vi "Main.vi"(8 "error in (no error)":errorcluster, 11 "DAQMH121119OrcaFlashBase in":refnum<class "DAQOrcaFlash.lvclass">) -> (0 "error out":errorcluster, 3 "component":refnum<class "DAQOrcaFlash.lvclass">)   [LabVIEW 2012, in "DAQOrcaFlash.lvclass"]
doc: "Main VI of the component."
uses:
  DAQOrcaFlash.lvclass
  binning.ctl
  visualisation_line_cluster.ctl
  merit_factor_type.ctl
  DAQOrcaFlash.lvclass/DAQOrcaFlash.ctl
  <vilib>/Distrio/Murmex/InitialiseMessage/InitialiseMessage.lvclass
  <vilib>/Distrio/Murmex/Murmex/command_enum.ctl
  <vilib>/Distrio/Murmex/TerminateMessage/TerminateMessage.lvclass
  <vilib>/Distrio/Murmex/StartMessage/StartMessage.lvclass
  <vilib>/Distrio/Murmex/StartMessage/run mode enum.ctl
  <vilib>/Distrio/Murmex/StopMessage/StopMessage.lvclass
  <vilib>/Distrio/Murmex/ConfigureMessage/ConfigureMessage.lvclass
  <vilib>/Distrio/Murmex/Murmex/update_cluster.ctl
  class variable.vi
  <vilib>/Distrio/Murmex/Murmex/Set VI reference.vi
  <vilib>/Distrio/Murmex/Murmex/Set configure at initialise.vi
  <vilib>/Distrio/Murmex/Murmex/Set relay start stop to observers.vi
  <vilib>/Distrio/Murmex/Murmex/Set log reference.vi
  <vilib>/Distrio/Murmex/Murmex/Set write log to disk.vi
  <vilib>/Distrio/Murmex/Murmex/Murmex.lvclass
  <vilib>/Distrio/Murmex/Message/Message.lvclass
panel:
  in  "button:configure":bool
  in  "button:quit":bool
  in  "terminate?":bool
  out "progress bar":sgl(slide) scale=0.0..1.0
  in  "Tab":T1(tab)
  in  "Rolling shutter pace":sgl[unit]=9.74436e-06 min=9.74436e-06 max=10 step=3.76e-09 format="%#_7g"
  out "Frames per second":dbl[unit]
  out "Virtual slit width":dbl[unit]
  in  "button:start_sweep":bool
  in  "y offset":u16 max=2048 step=4
  in  "x offset":u16 max=2048 step=4
  in  "y resolution":u16=2048 min=4 max=2048 step=4
  in  "x resolution":u16=2048 min=4 max=2048 step=4
  in  "binning":T2=1 items=["1x1"=1, "2x2"=2, "4x4"=4]
  in  "no. of frames":i32=1 min=1 step=1
  in  "line exposure time":dbl[unit]=0.1 caption="exposure time" min=9.700000000000001e-09 max=0.01
  in  "button:start focus":bool
  in  "wait b4 acquisition":dbl[unit]
  in  "file name":string
  in  "subfolder levels":string[](array[string])
  in  "Custom saving path":bool
  in  "directory out":path
  in  "button:convert":bool
  out "filename":string
  in  "directory in":path
  in  "ID":string="orca"
  in  "log":string
  out "time interval between MF":dbl
  out "Merit Factor":dbl
  in  "Merit factor type":T3
  in  "button:AO":bool
  in  "lines":T4[](array[typedef])
  in  "Conversion policy":T5={"Conversion Method"=10, "Minimum Value"=0, "Maximum Value"=0, "# Shifts"=0} {"Conversion Method" items=["Default"=10, "Most Significant Bits"=11, "Full Dynamic"=12, "Downshift"=13, "Given Range"=14, "90% Dynamic"=15, "Given Percent Range"=16]}
  # "Convert here properietary file formats of Hamamatsu to TIFF format."
  # "DAQOrcaFlash\n\nImplemented by:\nMarcel van 't Hoff\nLudovico Silvestri\nUniversity of Florence, Ital\n\nThis component supports only the Hamamatsu Orca Flash 4.0"
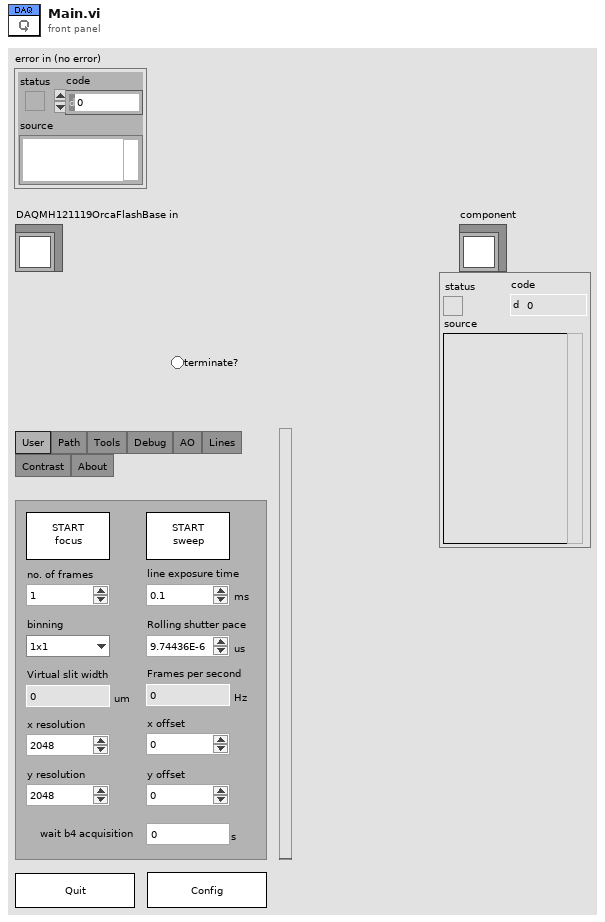
[diagram p1: front panel]
types:
  T1 = enum32{"User", "Path", "Tools", "Debug", "AO", "Lines", "Contrast", "About"}
  T2 = typedef "DAQOrcaFlash.lvclass/binning.ctl" = u16
  T3 = typedef "DAQOrcaFlash.lvclass/merit_factor_type.ctl" = enum16{"full frame intensity", "ROI beads", "Weber contrast", "Michelson contrast", "RMS contrast", "Line profile analysis", "ROI analysis", "FFT", "SNR", "5% brightest"}
  T4 = typedef "DAQOrcaFlash.lvclass/visualisation_line_cluster.ctl" = cluster{"direction":enum16{"horizontal", "vertical"}, "position":i32}
  T5 = cluster{"Conversion Method":u32, "Minimum Value":i32, "Maximum Value":i32, "# Shifts":i32}
  T6 = typedef "Murmex.lvlib/Murmex.lvclass/command_enum.ctl" = enum16{"null", "initialise", "reset", "terminate", "acknowledge", "update", "inspect", "inform", "proceed", "start", "stop", "fetch", "configure", "generic"}
  T7 = typedef "Murmex.lvlib/StartMessage.lvclass/run mode enum.ctl" = enum16{"infinite", "finite"}
  T8 = typedef "Murmex.lvlib/Murmex.lvclass/update_cluster.ctl" = cluster{"target ID":string, "key chains":string[], "values":variant[]}
  T9 = enum8{"Enabled", "Disabled", "Disabled and Grayed Out"}
  T10 = typedef "Murmex.lvclass/command_enum.ctl" = enum16{"null", "initialise", "reset", "terminate", "acknowledge", "update", "inspect", "inform", "proceed", "start", "stop", "fetch", "configure", "generic"}
  T11 = typedef "Murmex.lvclass/Event type enumerations.ctl" = enum16{"before", "after"}
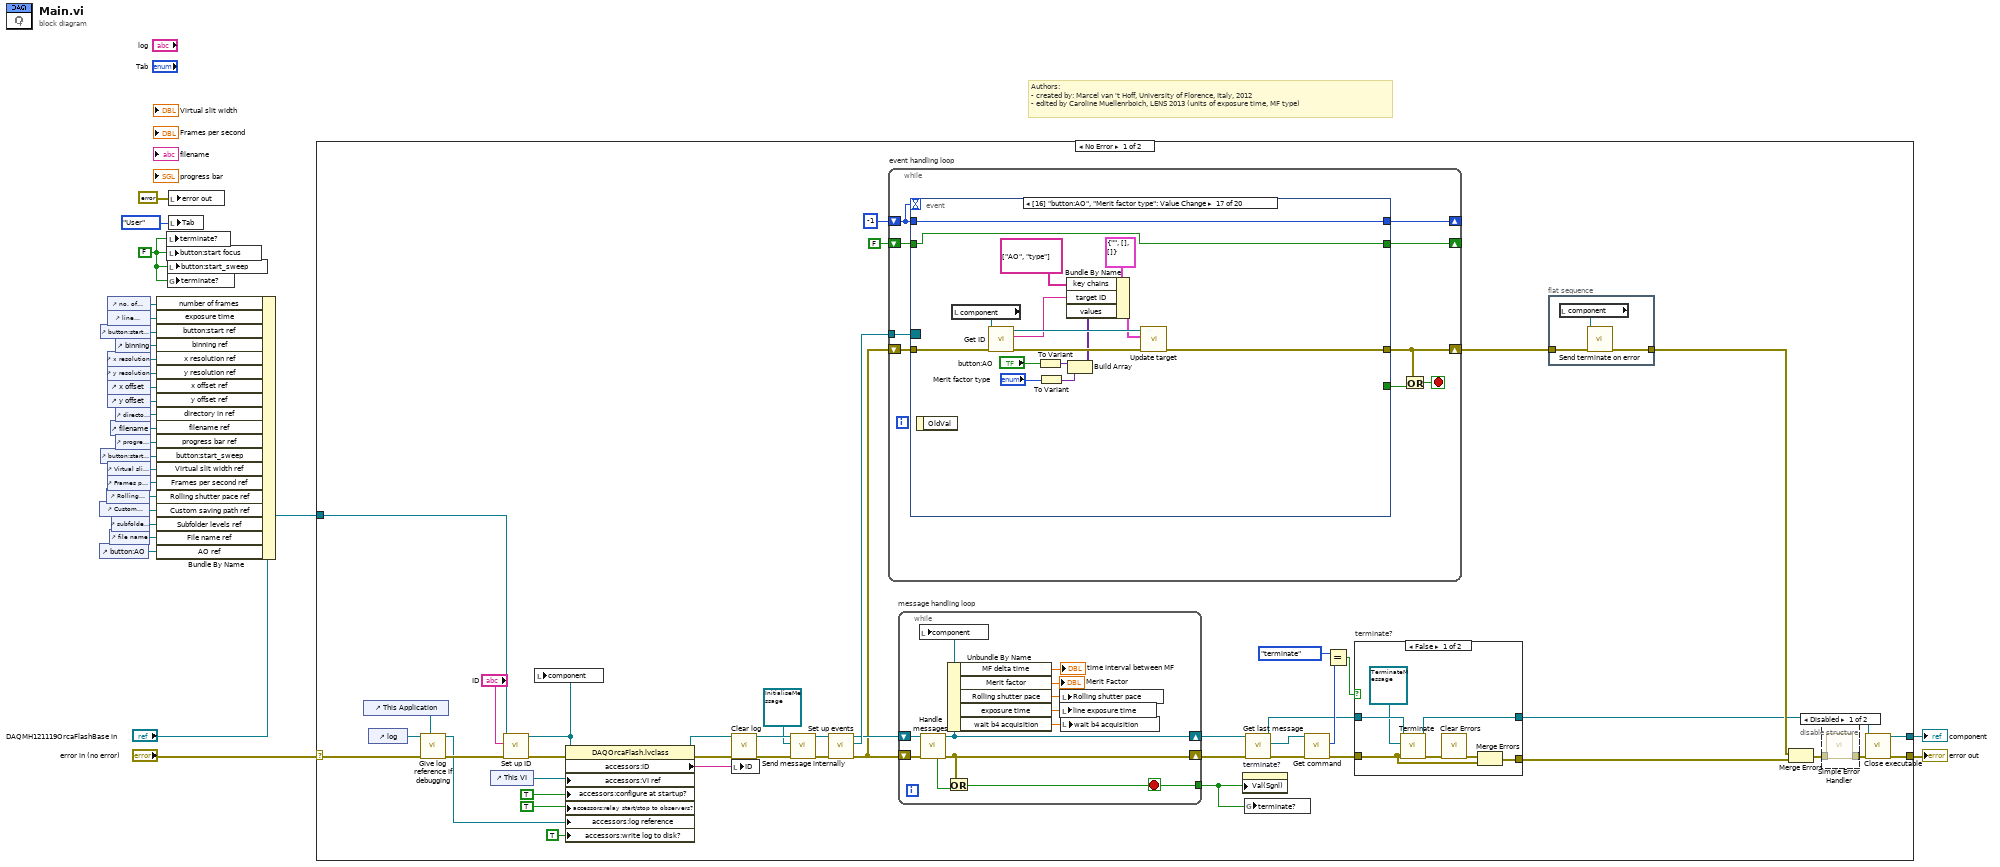
[diagram p0: block diagram]
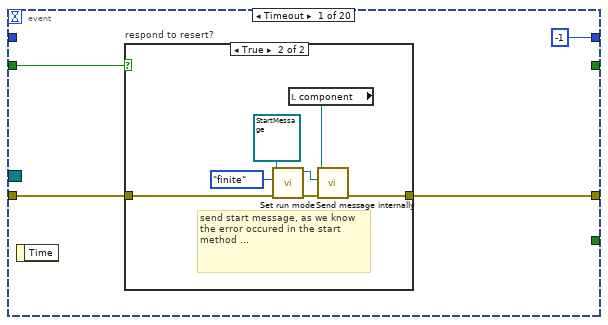
[diagram p4: hidden frame]
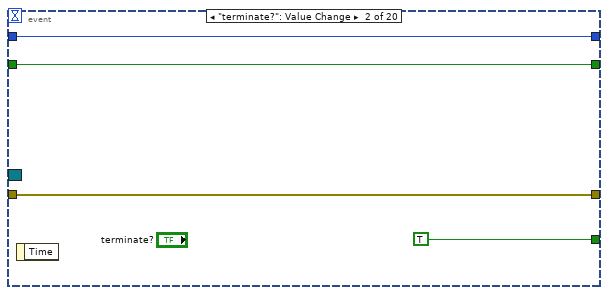
[diagram p6: hidden frame]
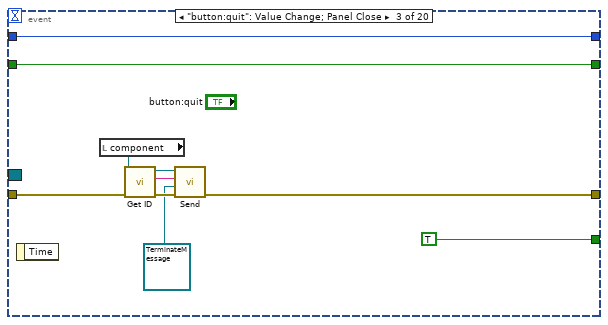
[diagram p7: hidden frame]
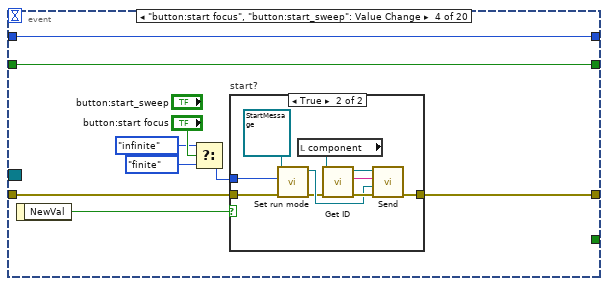
[diagram p8: hidden frame]
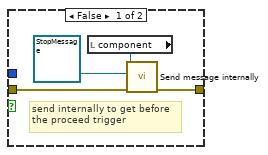
[diagram p9: hidden frame]
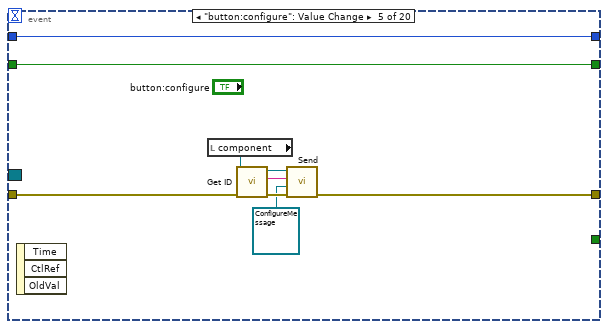
[diagram p10: hidden frame]
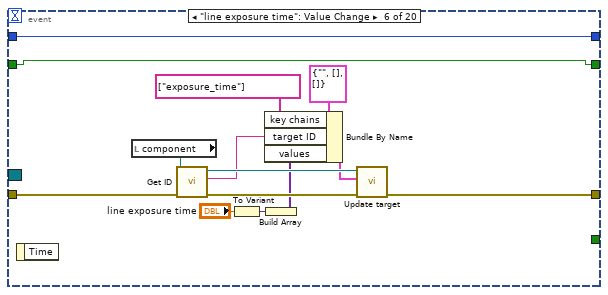
[diagram p11: hidden frame]
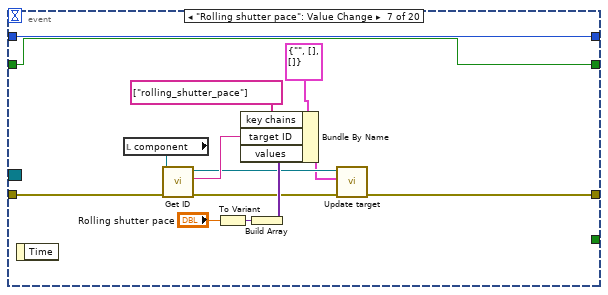
[diagram p12: hidden frame]
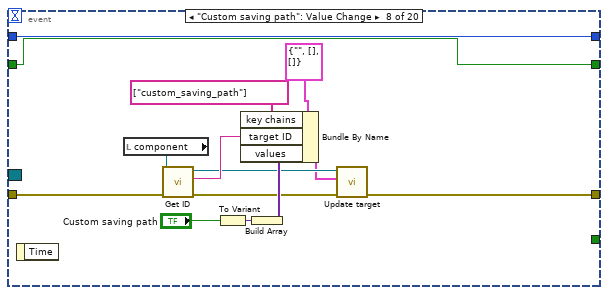
[diagram p13: hidden frame]
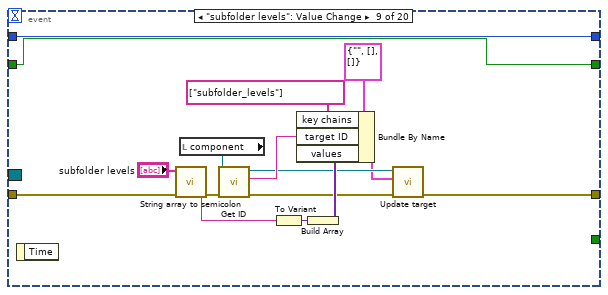
[diagram p14: hidden frame]
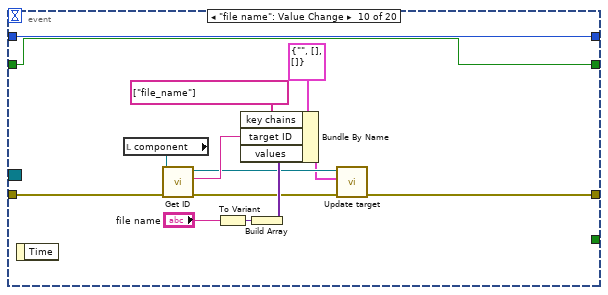
[diagram p15: hidden frame]
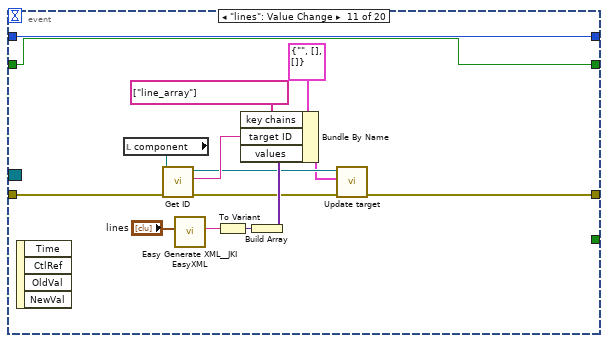
[diagram p16: hidden frame]
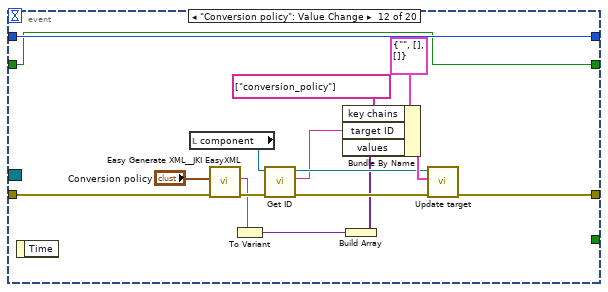
[diagram p17: hidden frame]
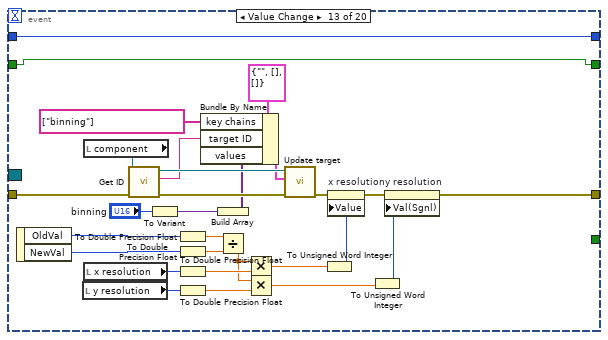
[diagram p18: hidden frame]
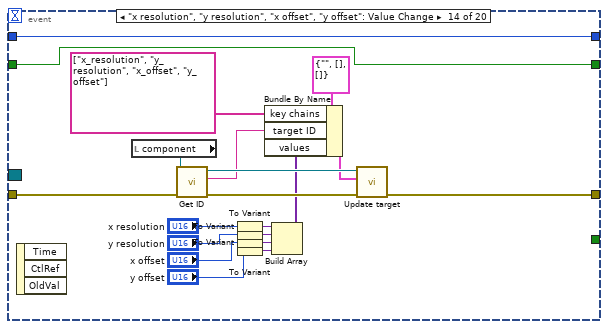
[diagram p19: hidden frame]
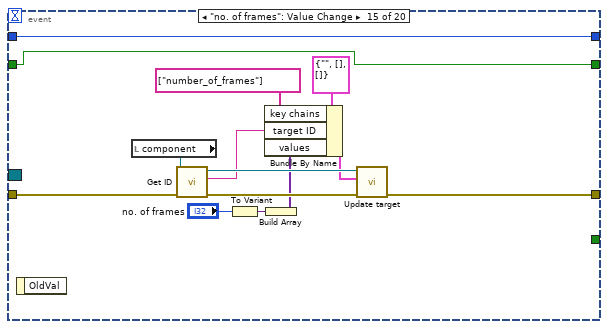
[diagram p20: hidden frame]
diagram:
  w9 = FALSE ("terminate?")
  # "Authors: \n- created by: Marcel van 't Hoff, University of Florence, Italy, 2012\n- edited by Caroline Muellenrboich, LENS 2013 (units of exposure time, MF type)"
  n1 = control-ref of="button:AO"() -> (w2:refnum<vi>)
  n2 = control-ref of="Custom saving path"() -> (w3:refnum<vi>)
  n3 = control-ref of="button:start focus"() -> (w20:refnum<vi>)
  n4 = control-ref of="button:start_sweep"() -> (w10:refnum<vi>)
  n5 = control-ref of="Rolling shutter pace"() -> (w6:refnum<vi>)
  n6 = control-ref of="no. of frames"() -> (w21:refnum<vi>)
  n7 = control-ref of="line exposure time"() -> (w22:refnum<vi>)
  n8 = control-ref of="x resolution"() -> (w18:refnum<vi>)
  n9 = control-ref of="y resolution"() -> (w17:refnum<vi>)
  n10 = control-ref of="x offset"() -> (w16:refnum<vi>)
  n11 = control-ref of="y offset"() -> (w15:refnum<vi>)
  n12 = control-ref of="Virtual slit width"() -> (w8:refnum<vi>)
  n13 = control-ref of="Frames per second"() -> (w7:refnum<vi>)
  n14 = control-ref of="file name"() -> (w5:refnum<vi>)
  n15 = control-ref of="filename"() -> (w13:refnum<vi>)
  n16 = control-ref of="subfolder levels"() -> (w4:refnum<vi>)
  n17 = control-ref of="binning"() -> (w19:refnum<vi>)
  n18 = control-ref of="directory in"() -> (w14:refnum<vi>)
  n19 = control-ref of="progress bar"() -> (w12:refnum<vi>)
  n20 = Bundle By Name(cluster="DAQMH121119OrcaFlashBase in", "number of frames"=w21, "exposure time"=w22, "button:start ref"=w20, "binning ref"=w19, "x resolution ref"=w18, "y resolution ref"=w17, "x offset ref"=w16, "y offset ref"=w15, "directory in ref"=w14, "filename ref"=w13, "progress bar ref"=w12, "button:start_sweep"=w10, "Virtual slit width ref"=w8, "Frames per second ref"=w7, "Rolling shutter pace ref"=w6, "Custom saving path ref"=w3, "Subfolder levels ref"=w4, "File name ref"=w5, "AO ref"=w2) -> (w23:refnum<class "DAQOrcaFlash.lvclass">)
  n21 = local write "terminate?"(w9) -> ()
  n22 = local write "button:start focus"(w9) -> ()
  n23 = local write "button:start_sweep"(w9) -> ()
  n24 = global write "class variable.vi" "terminate?"(w9) -> ()
  n25 = local write "error out"(errorcluster {"status"=FALSE, "code"=0, "source"=""} ("error out")) -> ()
  n26 = local write "Tab"(T1."User" ("Tab")) -> ()
  n27 = case shown="No Error" "error in (no error)" {
    selector: "error in (no error)" -> [w34 w437]
    tunnel: [w61 w437] -> w26
    tunnel: [w60 w436] -> w25
    tunnel: w23 -> [w66 w436]
    frame No Error {
      n28 = control-ref of="This Application"() -> (w30:refnum<vi>)
      n29 = control-ref of="log"() -> (w32:refnum<vi>)
      n30 = call "Give log reference if debugging.vi"("application ref"=w30, "error in (no error)"=w34, "log reference in"=w32) -> ("error out"=w33:errorcluster, "log reference out"=w31:refnum<vi>)  [unwired: 6 in, 1 out]
      n31 = control-ref of="This VI"() -> (w56:refnum<vi>)
      n32 = call <vilib>:"Set up ID.vi"("error in (no error)"=w33, "component ID"="ID", "MurmexBase in"=w66) -> ("error out"=w58:errorcluster, "MurmexBase out"=w47:refnum<class "DAQOrcaFlash.lvclass">)  [unwired: 6 in, 1 out]
      n33 = local write "component"(w47) -> ()
      n34 = property class="DAQOrcaFlash.lvclass"(reference=w47, error in=w58, "accessors:VI ref"=w56, "accessors:configure at startup?"=TRUE ("configure at startup?"), "accessors:relay start/stop to observers?"=TRUE ("relay start/stop to observers?"), "accessors:log reference"=w31, "accessors:write log to disk?"=TRUE ("write log to disk?")) -> (reference out=w54:refnum<class "DAQOrcaFlash.lvclass">, error out=w55:errorcluster, "accessors:ID"=w57:string)
      n35 = call <vilib>:"Clear log.vi"("error in (no error)"=w55, "MurmexBase in"=w54) -> ("error out"=w67:errorcluster, "MurmexBase out"=w71:refnum<class "DAQOrcaFlash.lvclass">)  [unwired: 8 in]
      n36 = local write "ID"(w57) -> ()
      n37 = call <vilib>:"Send message internally.vi"("error in (no error)"=w67, "Message"=refnum<class "InitialiseMessage.lvclass"> refnum ("Distrio Murmex 1.0:InitialiseMessage"), "Murmex in"=w71) -> ("error out"=w64:errorcluster, "Murmex out"=w63:refnum<class "DAQOrcaFlash.lvclass">)  [unwired: 7 in]
      n38 = call <vilib>:"Set up events.vi"("error in (no error)"=w64, "MurmexBase in"=w63) -> ("error out"=w36:errorcluster, "Event Registration Refnum"=w69:refnum<event-registration>, "MurmexBase out"=w38:refnum<class "DAQOrcaFlash.lvclass">)  [unwired: 7 in]
      n39 = while "event handling loop" {
        shift-right: [w94] -> _
        shift-left: -1 -> [w93]
        tunnel: w69 -> [w91]
        shift-right: [w90] -> w68
        shift-left: w36 -> [w92]
        shift-right: [w87] -> _
        shift-left: FALSE ("respond to reset?") -> [w86]
        stop <- w88 stop-if-true
        n40 = event shown="[16] \"button:AO\", \"Merit factor type\": Value Change" {
          selector: w91 -> [_ _ _ _ _ _ _ _ _ _ _ _ _ _ _ _ _ _ _ _]
          dyn-events: _ -> [_ _ _ _ _ _ _ _ _ _ _ _ _ _ _ _ _ _ _ _]
          timeout: w93 -> [_ _ _ _ _ _ _ _ _ _ _ _ _ _ _ _ _ _ _ _]
          tunnel: [-1 w110 w120 w129 w152 w166 w180 w194 w210 w224 w239 w255 w284 w304 w318 w332 w348 w350 w412 w424] -> w94
          tunnel: w93 -> [_ w110 w120 w129 w152 w166 w180 w194 w210 w224 w239 w255 w284 w304 w318 w332 w348 w355 w412 w424]
          tunnel: w92 -> [w96 w109 w113 w128 w148 w165 w179 w193 w199 w223 w238 w254 w283 w303 w317 w331 w347 w356 w410 w421]
          tunnel: [w95 w109 w115 w127 w147 w164 w172 w182 w203 w216 w231 w249 w266 w302 w316 w330 w336 w357 w409 w414] -> w90
          tunnel: [_ TRUE TRUE _ _ _ _ _ _ _ _ _ _ _ _ _ _ _ _ _] -> w89
          tunnel: [_ w107 w111 w121 w144 w153 w167 w181 w195 w211 w225 w240 w256 w285 w305 w319 w335 w352 w406 w413] -> w87
          tunnel: w86 -> [w97 w107 w111 w121 w144 w153 w167 w181 w195 w211 w225 w240 w256 w285 w305 w319 w335 w353 w406 w413]
          event Timeout {
            n41 = event-data() -> ()  [unwired: 1 in, 1 out]
            n42 = case "respond to resert?" shown="True" w97 {
              tunnel: w96 -> [w99 w102]
              tunnel: [w99 w106] -> w95
              frame False {
              }
              frame True {
                # "send start message, as we know the error occured in the start method ..."
                n43 = call <vilib>:"Set run mode.vi"("error in (no error)"=w102, "run mode"=run_mode_enum."finite", "StartMessage in"=refnum<class "StartMessage.lvclass"> refnum ("Distrio Murmex 1.0:StartMessage")) -> ("error out"=w101:errorcluster, "StartMessage out"=w103:refnum<class "StartMessage.lvclass">)  [unwired: 7 in]
                n44 = local read "component"() -> (w105:refnum<class "DAQOrcaFlash.lvclass">)
                n45 = call <vilib>:"Send message internally.vi"("error in (no error)"=w101, "Message"=w103, "Murmex in"=w105) -> ("error out"=w106:errorcluster)  [unwired: 7 in, 1 out]
              }
            }
          }
          event "terminate?": Value Change {
            n46 = event-data() -> ()  [unwired: 1 in, 1 out]
          }
          event "button:quit": Value Change; Panel Close {
            n47 = event-data() -> ()  [unwired: 1 in, 1 out]
            n48 = local read "component"() -> (w118:refnum<class "DAQOrcaFlash.lvclass">)
            n49 = call <vilib>:"Get ID.vi"("error in (no error)"=w113, "Murmex in"=w118) -> ("error out"=w114:errorcluster, "component id"=w116:string, "Murmex out"=w117:refnum<class "DAQOrcaFlash.lvclass">)  [unwired: 7 in]
            n50 = call <vilib>:"Send.vi"("error in (no error)"=w114, "Message"=refnum<class "TerminateMessage.lvclass"> refnum ("Message in"), "recipient"=w116, "Murmex in"=w117) -> ("error out"=w115:errorcluster)  [unwired: 6 in, 1 out]
          }
          event "button:start focus", "button:start_sweep": Value Change {
            n51 = event-data() -> ("NewVal"=w124:bool)  [unwired: 1 in]
            n52 = Select(t=run_mode_enum."infinite" ("run mode"), s="button:start focus", f=run_mode_enum."finite" ("run mode")) -> (s? t:f=w125:T7)
            n53 = case "start?" shown="True" w124 {
              tunnel: [w132 w139] -> w127
              tunnel: w128 -> [w133 w136]
              tunnel: w125 -> [_ w134]
              frame False {
                # "send internally to get before\nthe proceed trigger"
                n54 = local read "component"() -> (w131:refnum<class "DAQOrcaFlash.lvclass">)
                n55 = call <vilib>:"Send message internally.vi"("error in (no error)"=w133, "Message"=refnum<class "StopMessage.lvclass"> refnum ("Distrio Murmex 1.0:StopMessage"), "Murmex in"=w131) -> ("error out"=w132:errorcluster)  [unwired: 7 in, 1 out]
              }
              frame True {
                n56 = call <vilib>:"Set run mode.vi"("error in (no error)"=w136, "run mode"=w134, "StartMessage in"=refnum<class "StartMessage.lvclass"> refnum ("Distrio Murmex 1.0:StartMessage")) -> ("error out"=w135:errorcluster, "StartMessage out"=w137:refnum<class "StartMessage.lvclass">)  [unwired: 7 in]
                n57 = local read "component"() -> (w143:refnum<class "DAQOrcaFlash.lvclass">)
                n58 = call <vilib>:"Get ID.vi"("error in (no error)"=w135, "Murmex in"=w143) -> ("error out"=w140:errorcluster, "component id"=w141:string, "Murmex out"=w142:refnum<class "DAQOrcaFlash.lvclass">)  [unwired: 7 in]
                n59 = call <vilib>:"Send.vi"("error in (no error)"=w140, "Message"=w137, "recipient"=w141, "Murmex in"=w142) -> ("error out"=w139:errorcluster)  [unwired: 6 in, 1 out]
              }
            }
          }
          event "button:configure": Value Change {
            n60 = event-data() -> ()  [unwired: 1 in, 3 out]
            n61 = local read "component"() -> (w146:refnum<class "DAQOrcaFlash.lvclass">)
            n62 = call <vilib>:"Get ID.vi"("error in (no error)"=w148, "Murmex in"=w146) -> ("error out"=w149:errorcluster, "component id"=w150:string, "Murmex out"=w151:refnum<class "DAQOrcaFlash.lvclass">)  [unwired: 7 in]
            n63 = call <vilib>:"Send.vi"("error in (no error)"=w149, "Message"=refnum<class "ConfigureMessage.lvclass"> refnum ("ConfigureMessage"), "recipient"=w150, "Murmex in"=w151) -> ("error out"=w147:errorcluster)  [unwired: 6 in, 1 out]
          }
          event "line exposure time": Value Change {
            n64 = event-data() -> ()  [unwired: 1 in, 1 out]
            n65 = local read "component"() -> (w163:refnum<class "DAQOrcaFlash.lvclass">)
            n66 = call <vilib>:"Get ID.vi"("error in (no error)"=w165, "Murmex in"=w163) -> ("error out"=w161:errorcluster, "component id"=w158:string, "Murmex out"=w162:refnum<class "DAQOrcaFlash.lvclass">)  [unwired: 7 in]
            n67 = To Variant(anything="line exposure time") -> (Variant=w156:variant)
            n68 = Build Array(w156) -> (w155:variant[])
            n69 = Bundle By Name(cluster=T8 {"target ID"="", "key chains"=[], "values"=[]} ("update cluster"), "key chains"=string[] ["exposure_time"], "target ID"=w158, "values"=w155) -> (w159:T8)
            n70 = call <vilib>:"Update target.vi"("error in (no error)"=w161, "update cluster"=w159, "MurmexBase in"=w162) -> ("error out"=w164:errorcluster)  [unwired: 7 in, 1 out]
          }
          event "Rolling shutter pace": Value Change {
            n71 = event-data() -> ()  [unwired: 1 in, 1 out]
            n72 = local read "component"() -> (w177:refnum<class "DAQOrcaFlash.lvclass">)
            n73 = call <vilib>:"Get ID.vi"("error in (no error)"=w179, "Murmex in"=w177) -> ("error out"=w173:errorcluster, "component id"=w176:string, "Murmex out"=w171:refnum<class "DAQOrcaFlash.lvclass">)  [unwired: 7 in]
            n74 = To Variant(anything="Rolling shutter pace") -> (Variant=w178:variant)
            n75 = Build Array(w178) -> (w174:variant[])
            n76 = Bundle By Name(cluster=T8 {"target ID"="", "key chains"=[], "values"=[]} ("update cluster"), "key chains"=string[] ["rolling_shutter_pace"], "target ID"=w176, "values"=w174) -> (w169:T8)
            n77 = call <vilib>:"Update target.vi"("error in (no error)"=w173, "update cluster"=w169, "MurmexBase in"=w171) -> ("error out"=w172:errorcluster)  [unwired: 7 in, 1 out]
          }
          event "Custom saving path": Value Change {
            n78 = event-data() -> ()  [unwired: 1 in, 1 out]
            n79 = local read "component"() -> (w191:refnum<class "DAQOrcaFlash.lvclass">)
            n80 = call <vilib>:"Get ID.vi"("error in (no error)"=w193, "Murmex in"=w191) -> ("error out"=w187:errorcluster, "component id"=w190:string, "Murmex out"=w186:refnum<class "DAQOrcaFlash.lvclass">)  [unwired: 7 in]
            n81 = To Variant(anything="Custom saving path") -> (Variant=w192:variant)
            n82 = Build Array(w192) -> (w188:variant[])
            n83 = Bundle By Name(cluster=T8 {"target ID"="", "key chains"=[], "values"=[]} ("update cluster"), "key chains"=string[] ["custom_saving_path"], "target ID"=w190, "values"=w188) -> (w184:T8)
            n84 = call <vilib>:"Update target.vi"("error in (no error)"=w187, "update cluster"=w184, "MurmexBase in"=w186) -> ("error out"=w182:errorcluster)  [unwired: 7 in, 1 out]
          }
          event "subfolder levels": Value Change {
            n85 = event-data() -> ()  [unwired: 1 in, 1 out]
            n86 = call "String array to semicolon.vi"("error in"=w199, "String array"="subfolder levels") -> ("error out"=w198:errorcluster, "Semicolon string"=w197:string)  [unwired: 8 in]
            n87 = local read "component"() -> (w208:refnum<class "DAQOrcaFlash.lvclass">)
            n88 = call <vilib>:"Get ID.vi"("error in (no error)"=w198, "Murmex in"=w208) -> ("error out"=w204:errorcluster, "component id"=w207:string, "Murmex out"=w202:refnum<class "DAQOrcaFlash.lvclass">)  [unwired: 7 in]
            n89 = To Variant(anything=w197) -> (Variant=w209:variant)
            n90 = Build Array(w209) -> (w205:variant[])
            n91 = Bundle By Name(cluster=T8 {"target ID"="", "key chains"=[], "values"=[]} ("update cluster"), "key chains"=string[] ["subfolder_levels"], "target ID"=w207, "values"=w205) -> (w200:T8)
            n92 = call <vilib>:"Update target.vi"("error in (no error)"=w204, "update cluster"=w200, "MurmexBase in"=w202) -> ("error out"=w203:errorcluster)  [unwired: 7 in, 1 out]
          }
          event "file name": Value Change {
            n93 = event-data() -> ()  [unwired: 1 in, 1 out]
            n94 = local read "component"() -> (w221:refnum<class "DAQOrcaFlash.lvclass">)
            n95 = call <vilib>:"Get ID.vi"("error in (no error)"=w223, "Murmex in"=w221) -> ("error out"=w217:errorcluster, "component id"=w220:string, "Murmex out"=w215:refnum<class "DAQOrcaFlash.lvclass">)  [unwired: 7 in]
            n96 = To Variant(anything="file name") -> (Variant=w222:variant)
            n97 = Build Array(w222) -> (w218:variant[])
            n98 = Bundle By Name(cluster=T8 {"target ID"="", "key chains"=[], "values"=[]} ("update cluster"), "key chains"=string[] ["file_name"], "target ID"=w220, "values"=w218) -> (w213:T8)
            n99 = call <vilib>:"Update target.vi"("error in (no error)"=w217, "update cluster"=w213, "MurmexBase in"=w215) -> ("error out"=w216:errorcluster)  [unwired: 7 in, 1 out]
          }
          event "lines": Value Change {
            n100 = event-data() -> ()  [unwired: 1 in, 4 out]
            n101 = local read "component"() -> (w236:refnum<class "DAQOrcaFlash.lvclass">)
            n102 = call <vilib>:"Get ID.vi"("error in (no error)"=w238, "Murmex in"=w236) -> ("error out"=w232:errorcluster, "component id"=w235:string, "Murmex out"=w230:refnum<class "DAQOrcaFlash.lvclass">)  [unwired: 7 in]
            n103 = call <vilib>:"Easy Generate XML__JKI EasyXML.vi"("LabVIEW Data"="lines") -> ("XML String"=w226:string)  [unwired: 9 in, 1 out]
            n104 = To Variant(anything=w226) -> (Variant=w237:variant)
            n105 = Build Array(w237) -> (w233:variant[])
            n106 = Bundle By Name(cluster=T8 {"target ID"="", "key chains"=[], "values"=[]} ("update cluster"), "key chains"=string[] ["line_array"], "target ID"=w235, "values"=w233) -> (w228:T8)
            n107 = call <vilib>:"Update target.vi"("error in (no error)"=w232, "update cluster"=w228, "MurmexBase in"=w230) -> ("error out"=w231:errorcluster)  [unwired: 7 in, 1 out]
          }
          event "Conversion policy": Value Change {
            n108 = event-data() -> ()  [unwired: 1 in, 1 out]
            n109 = local read "component"() -> (w250:refnum<class "DAQOrcaFlash.lvclass">)
            n110 = call <vilib>:"Easy Generate XML__JKI EasyXML.vi"("error in (no error)"=w254, "LabVIEW Data"="Conversion policy") -> ("error out"=w253:errorcluster, "XML String"=w242:string)  [unwired: 8 in]
            n111 = To Variant(anything=w242) -> (Variant=w243:variant)
            n112 = call <vilib>:"Get ID.vi"("error in (no error)"=w253, "Murmex in"=w250) -> ("error out"=w251:errorcluster, "component id"=w244:string, "Murmex out"=w245:refnum<class "DAQOrcaFlash.lvclass">)  [unwired: 7 in]
            n113 = Build Array(w243) -> (w241:variant[])
            n114 = Bundle By Name(cluster=T8 {"target ID"="", "key chains"=[], "values"=[]} ("update cluster"), "key chains"=string[] ["conversion_policy"], "target ID"=w244, "values"=w241) -> (w246:T8)
            n115 = call <vilib>:"Update target.vi"("error in (no error)"=w251, "update cluster"=w246, "MurmexBase in"=w245) -> ("error out"=w249:errorcluster)  [unwired: 7 in, 1 out]
          }
          event Value Change {
            n116 = event-data() -> ("OldVal"=w261:T2, "NewVal"=w260:T2)  [unwired: 1 in]
            n117 = local read "y resolution"() -> (w274:u16)
            n118 = local read "component"() -> (w282:refnum<class "DAQOrcaFlash.lvclass">)
            n119 = local read "x resolution"() -> (w273:u16)
            n120 = call <vilib>:"Get ID.vi"("error in (no error)"=w283, "Murmex in"=w282) -> ("error out"=w280:errorcluster, "component id"=w277:string, "Murmex out"=w281:refnum<class "DAQOrcaFlash.lvclass">)  [unwired: 7 in]
            n121 = To Variant(anything="binning") -> (Variant=w269:variant)
            n122 = To Double Precision Float(number=w261) -> (double precision float=w259:dbl)
            n123 = To Double Precision Float(number=w260) -> (double precision float=w258:dbl)
            n124 = To Double Precision Float(number=w273) -> (double precision float=w270:dbl)
            n125 = To Double Precision Float(number=w274) -> (double precision float=w271:dbl)
            n126 = Build Array(w269) -> (w275:variant[])
            n127 = Bundle By Name(cluster=T8 {"target ID"="", "key chains"=[], "values"=[]} ("update cluster"), "key chains"=string[] ["binning"], "target ID"=w277, "values"=w275) -> (w278:T8)
            n128 = Divide(x=w259, y=w258) -> (x/y=w257:dbl)
            n129 = Multiply(x=w257, y=w270) -> (x*y=w267:dbl)
            n130 = Multiply(x=w257, y=w271) -> (x*y=w268:dbl)
            n131 = call <vilib>:"Update target.vi"("error in (no error)"=w280, "update cluster"=w278, "MurmexBase in"=w281) -> ("error out"=w265:errorcluster)  [unwired: 7 in, 1 out]
            n132 = To Unsigned Word Integer(number=w267) -> (unsigned 16bit integer=w264:u16)
            n133 = property on="x resolution" class="DigNum (strict)"(error in=w265, "Value"=w264) -> (error out=w262:errorcluster)  [unwired: 1 in, 1 out]
            n134 = To Unsigned Word Integer(number=w268) -> (unsigned 16bit integer=w263:u16)
            n135 = property on="y resolution" class="DigNum (strict)"(error in=w262, "Val(Sgnl)"=w263) -> (error out=w266:errorcluster)  [unwired: 1 in, 1 out]
          }
          event "x resolution", "y resolution", "x offset", "y offset": Value Change {
            n136 = event-data() -> ()  [unwired: 1 in, 3 out]
            n137 = local read "component"() -> (w301:refnum<class "DAQOrcaFlash.lvclass">)
            n138 = call <vilib>:"Get ID.vi"("error in (no error)"=w303, "Murmex in"=w301) -> ("error out"=w299:errorcluster, "component id"=w296:string, "Murmex out"=w300:refnum<class "DAQOrcaFlash.lvclass">)  [unwired: 7 in]
            n139 = To Variant(anything="x resolution") -> (Variant=w289:variant)
            n140 = To Variant(anything="y resolution") -> (Variant=w288:variant)
            n141 = To Variant(anything="x offset") -> (Variant=w287:variant)
            n142 = To Variant(anything="y offset") -> (Variant=w286:variant)
            n143 = Build Array(w289, w288, w287, w286) -> (w290:variant[])
            n144 = Bundle By Name(cluster=T8 {"target ID"="", "key chains"=[], "values"=[]} ("update cluster"), "key chains"=string[] ["x_resolution", "y_resolution", "x_offset", "y_offset"], "target ID"=w296, "values"=w290) -> (w297:T8)
            n145 = call <vilib>:"Update target.vi"("error in (no error)"=w299, "update cluster"=w297, "MurmexBase in"=w300) -> ("error out"=w302:errorcluster)  [unwired: 7 in, 1 out]
          }
          event "no. of frames": Value Change {
            n146 = event-data() -> ()  [unwired: 1 in, 1 out]
            n147 = local read "component"() -> (w315:refnum<class "DAQOrcaFlash.lvclass">)
            n148 = call <vilib>:"Get ID.vi"("error in (no error)"=w317, "Murmex in"=w315) -> ("error out"=w313:errorcluster, "component id"=w310:string, "Murmex out"=w314:refnum<class "DAQOrcaFlash.lvclass">)  [unwired: 7 in]
            n149 = To Variant(anything="no. of frames") -> (Variant=w306:variant)
            n150 = Build Array(w306) -> (w308:variant[])
            n151 = Bundle By Name(cluster=T8 {"target ID"="", "key chains"=[], "values"=[]} ("update cluster"), "key chains"=string[] ["number_of_frames"], "target ID"=w310, "values"=w308) -> (w311:T8)
            n152 = call <vilib>:"Update target.vi"("error in (no error)"=w313, "update cluster"=w311, "MurmexBase in"=w314) -> ("error out"=w316:errorcluster)  [unwired: 7 in, 1 out]
          }
          event "wait b4 acquisition": Value Change {
            # "waitb4 is a fun name for a control, but do you really need\nto use this also for the settings?"
            n153 = event-data() -> ()  [unwired: 1 in, 1 out]
            n154 = local read "component"() -> (w329:refnum<class "DAQOrcaFlash.lvclass">)
            n155 = call <vilib>:"Get ID.vi"("error in (no error)"=w331, "Murmex in"=w329) -> ("error out"=w327:errorcluster, "component id"=w324:string, "Murmex out"=w328:refnum<class "DAQOrcaFlash.lvclass">)  [unwired: 7 in]
            n156 = To Variant(anything="wait b4 acquisition") -> (Variant=w321:variant)
            n157 = Build Array(w321) -> (w322:variant[])
            n158 = Bundle By Name(cluster=T8 {"target ID"="", "key chains"=[], "values"=[]} ("update cluster"), "key chains"=string[] ["waitb4"], "target ID"=w324, "values"=w322) -> (w325:T8)
            n159 = call <vilib>:"Update target.vi"("error in (no error)"=w327, "update cluster"=w325, "MurmexBase in"=w328) -> ("error out"=w330:errorcluster)  [unwired: 7 in, 1 out]
          }
          event "button:AO": Value Change {
            n160 = event-data() -> ()  [unwired: 1 in, 1 out]
            n161 = local read "component"() -> (w346:refnum<class "DAQOrcaFlash.lvclass">)
            n162 = call <vilib>:"Get ID.vi"("error in (no error)"=w347, "Murmex in"=w346) -> ("error out"=w344:errorcluster, "component id"=w337:string, "Murmex out"=w345:refnum<class "DAQOrcaFlash.lvclass">)  [unwired: 7 in]
            n163 = To Variant(anything="button:AO") -> (Variant=w339:variant)
            n164 = To Variant(anything="Merit factor type") -> (Variant=w334:variant)
            n165 = Build Array(w339, w334) -> (w340:variant[])
            n166 = Bundle By Name(cluster=T8 {"target ID"="", "key chains"=[], "values"=[]} ("update cluster"), "key chains"=string[] ["AO", "type"], "target ID"=w337, "values"=w340) -> (w342:T8)
            n167 = call <vilib>:"Update target.vi"("error in (no error)"=w344, "update cluster"=w342, "MurmexBase in"=w345) -> ("error out"=w336:errorcluster)  [unwired: 7 in, 1 out]
          }
          event User Event {
            w349 = 5000  # wait for starting
            n168 = event-data() -> ("command"=w358:T10, "event type"=w354:T11)  [unwired: 1 in]
            n169 = case "command?" shown="\"reset\"" w358 {
              tunnel: [w363 w375 w387 w402 w405] -> w357
              tunnel: w356 -> [w362 w374 w388 w402 w405]
              tunnel: [w361 w373 w386 w400 w404] -> w351
              tunnel: w355 -> [w361 w373 w385 w400 w404]
              tunnel: w354 -> [w360 w372 w384 _ _]
              tunnel: [w359 w371 w383 w401 w403] -> w352
              tunnel: w353 -> [w359 w371 w383 _ w403]
              frame "stop" {
                n170 = case shown="\"after\"" w360 {
                  tunnel: [w364 w370] -> w363
                  tunnel: w362 -> [w364 w367]
                  frame "before", Default {
                  }
                  frame "after" {
                    n171 = local read "component"() -> (w368:refnum<class "DAQOrcaFlash.lvclass">)
                    n172 = call "Get GUI refs.vi"("error in (no error)"=w367, "DAQMH121119OrcaFlash in"=w368) -> ("error out"=w366:errorcluster, "Array"=w365:refnum<vi>[])  [unwired: 7 in, 1 out]
                    n173 = call <vilib>:"Disable GUI elements.vi"("error in (no error)"=w366, "enabled state"=T9."Enabled", "control refs"=w365) -> ("error out"=w370:errorcluster)  [unwired: 8 in]
                  }
                }
              }
              frame "start" {
                n174 = case shown="\"after\"" w372 {
                  tunnel: [w376 w382] -> w375
                  tunnel: w374 -> [w376 w380]
                  frame "before", Default {
                  }
                  frame "after" {
                    n175 = local read "component"() -> (w377:refnum<class "DAQOrcaFlash.lvclass">)
                    n176 = call "Get GUI refs.vi"("error in (no error)"=w380, "DAQMH121119OrcaFlash in"=w377) -> ("error out"=w379:errorcluster, "Array"=w378:refnum<vi>[])  [unwired: 7 in, 1 out]
                    n177 = call <vilib>:"Disable GUI elements.vi"("error in (no error)"=w379, "enabled state"=T9."Disabled and Grayed Out", "control refs"=w378) -> ("error out"=w382:errorcluster)  [unwired: 8 in]
                  }
                }
              }
              frame "initialise" {
                n178 = case shown="\"before\", Default" w384 {
                  tunnel: w388 -> [w390 w398]
                  tunnel: [w389 w397] -> w387
                  tunnel: [w395 -1] -> w386
                  tunnel: w385 -> [w395 _]
                  frame "before", Default {
                    n179 = local read "component"() -> (w391:refnum<class "DAQOrcaFlash.lvclass">)
                    n180 = call "Get GUI refs.vi"("error in (no error)"=w390, "DAQMH121119OrcaFlash in"=w391) -> ("error out"=w393:errorcluster, "Array"=w392:refnum<vi>[])  [unwired: 7 in, 1 out]
                    n181 = call <vilib>:"Disable GUI elements.vi"("error in (no error)"=w393, "enabled state"=T9."Disabled and Grayed Out", "control refs"=w392) -> ("error out"=w389:errorcluster)  [unwired: 8 in]
                  }
                  frame "after" {
                    n182 = local read "component"() -> (w399:refnum<class "DAQOrcaFlash.lvclass">)
                    n183 = call "Initialise parameters.vi"("error in (no error)"=w398, "DAQMH121119OrcaFlash in"=w399) -> ("error out"=w397:errorcluster)  [unwired: 8 in, 1 out]
                  }
                }
              }
              frame "reset" {
                w401 = TRUE  # respond to reset?
              }
              frame Default {
              }
            }
            n184 = Select(t=w349, s=w352, f=w351) -> (s? t:f=w350:i32)
          }
          event "button:convert": Value Change {
            n185 = event-data() -> ()  [unwired: 1 in, 1 out]
            n186 = local read "component"() -> (w411:refnum<class "DAQOrcaFlash.lvclass">)
            n187 = call "Convert directory new.vi"("error in (no error)"=w410, "directory out"="directory out", "directory in"="directory in", "DAQOrcaFlash in"=w411) -> ("error out"=w409:errorcluster)  [unwired: 6 in, 1 out]
          }
          event "directory in", "directory out": Value Change {
            n188 = event-data() -> ()  [unwired: 1 in, 1 out]
            n189 = local read "directory out"() -> (w423:path)
            n190 = local read "directory in"() -> (w420:path)
            n191 = call <vilib>:"Check if File or Folder Exists.vi"("error in (no error)"=w421, "path"=w423) -> ("error out"=w422:errorcluster, "file or folder exists?"=w418:bool)  [unwired: 7 in, 1 out]
            n192 = call <vilib>:"Check if File or Folder Exists.vi"("error in (no error)"=w422, "path"=w420) -> ("error out"=w415:errorcluster, "file or folder exists?"=w419:bool)  [unwired: 7 in, 1 out]
            n193 = And(x=w419, y=w418) -> (x .and. y?=w417:bool)
            n194 = call "bool_to_enable_state.vi"("boolean in"=w417) -> ("enabled status out"=w416:T9)  [unwired: 4 in]
            n195 = property on="button:convert" class="Bool"(error in=w415, "DisabledEnum"=w416) -> (error out=w414:errorcluster)  [unwired: 1 in, 1 out]
          }
        }
        n196 = Or(x=w90, y=w89) -> (x .or. y?=w88:bool)
      }
      n197 = while "message handling loop" {
        shift-right: [w431] -> w44
        shift-left: w36 -> [w433]
        shift-right: [w430] -> w46
        shift-left: w38 -> [w435]
        tunnel: [w432] -> w37
        stop <- w432 stop-if-true
        n198 = call <vilib>:"Handle messages.vi"("error in (no error)"=w433, "Murmex in"=w435) -> ("error out"=w431:errorcluster, "Murmex out"=w430:refnum<class "DAQOrcaFlash.lvclass">, "terminated?"=w434:bool)  [unwired: 7 in]
        n199 = local write "component"(w430) -> ()
        n200 = Or(x=w431, y=w434) -> (x .or. y?=w432:bool)
        n201 = Unbundle By Name(w430) -> ("MF delta time"=→"time interval between MF":dbl, "Merit factor"=→"Merit Factor":dbl, "Rolling shutter pace"=w429:sgl[unit], "exposure time"=w428:dbl[unit], "wait b4 acquisition"=w427:dbl[unit])
        n202 = local write "Rolling shutter pace"(w429) -> ()
        n203 = local write "line exposure time"(w428) -> ()
        n204 = local write "wait b4 acquisition"(w427) -> ()
      }
      n205 = property on="terminate?" class="Bool (strict)"("Val(Sgnl)"=w37) -> ()  [unwired: 2 in, 2 out]
      n206 = global write "class variable.vi" "terminate?"(w37) -> ()
      n207 = call <vilib>:"Get last message.vi"("error in (no error)"=w44, "MurmexBase in"=w46) -> ("error out"=w43:errorcluster, "Message"=w42:refnum<class "Message.lvclass">, "MurmexBase out"=w45:refnum<class "DAQOrcaFlash.lvclass">)  [unwired: 7 in]
      n208 = call <vilib>:"Get command.vi"("error in (no error)"=w43, "Message in"=w42) -> ("error out"=w50:errorcluster, "command"=w52:T6)  [unwired: 7 in, 1 out]
      n209 = Equal?(x=command_enum."terminate", y=w52) -> (x = y?=w48:bool)
      n210 = case "terminate?" shown="False" w48 {
        tunnel: w45 -> [w79 w82]
        tunnel: [w78 w82] -> w59
        tunnel: w50 -> [w77 w81]
        tunnel: [w75 w81] -> w49
        frame False {
          n211 = call-dynamic "Terminate.vi"("error in (no error)"=w77, "Message in"=refnum<class "TerminateMessage.lvclass"> refnum, "DAQMH121119OrcaFlash in"=w79) -> ("error out"=w80:errorcluster, "DAQMH121119OrcaFlash out"=w78:refnum<class "DAQOrcaFlash.lvclass">)  [unwired: 7 in]
          n212 = call <vilib>:"Clear Errors.vi"("error in (no error)"=w80) -> ("error out"=w76:errorcluster)  [unwired: 6 in]
          n213 = Merge Errors(w76, w77) -> (w75:errorcluster)
        }
        frame True {
        }
      }
      n214 = flat-sequence {
        tunnel: w68 -> [w85]
        tunnel: [w83] -> w62
        frame #0 {
          n215 = local read "component"() -> (w84:refnum<class "DAQOrcaFlash.lvclass">)
          n216 = call <vilib>:"Send terminate on error.vi"("error in (no error)"=w85, "Murmex in"=w84) -> ("error out"=w83:errorcluster)  [unwired: 8 in, 1 out]
        }
      }
      n217 = Merge Errors(w62, w49) -> (w40:errorcluster)
      n218 = disable-structure shown="Disabled" {
        disable-tunnel: w40 -> [w73 _]
        disable-tunnel: [w72 _] -> w39
        frame Disabled {
          n219 = call <vilib>:"Simple Error Handler.vi"("error in (no error)"=w73) -> ("error out"=w72:errorcluster)  [unwired: 4 in, 4 out]
        }
        frame Enabled {
        }
      }
      n220 = call <vilib>:"Close executable.vi"("error in (no error)"=w39, "MurmexBase in"=w59) -> ("error out"=w61:errorcluster, "MurmexBase out"=w60:refnum<class "DAQOrcaFlash.lvclass">)  [unwired: 8 in]
    }
    frame Error {
    }
  }
  "error out" <- w26
  "component" <- w25
